vi "EpochConverter_old.vi"(11 "Epoch time":u32) -> (0 "Date":string, 3 "String":string)   [LabVIEW 2015]
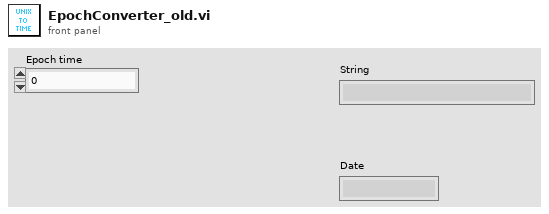
[diagram p1: front panel]
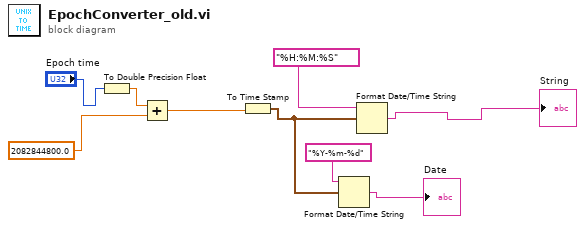
[diagram p0: block diagram]
diagram:
  n1 = To Double Precision Float(number="Epoch time") -> (double precision float=w6:dbl)
  n2 = Add(x=w6, y=2082844800.0) -> (x+y=w8:dbl)
  n3 = To Time Stamp(1:w8) -> (0:w3:timestamp)
  n4 = Format Date/Time String(time format string (%c)="%Y-%m-%d", seconds (now)=w3) -> (date/time string=→"Date":string)  [unwired: 1 in]
  n5 = Format Date/Time String(time format string (%c)="%H:%M:%S", seconds (now)=w3) -> (date/time string=→"String":string)  [unwired: 1 in]
